vi "Show Recipe.vi"(8 "error in (no error)":errorcluster, 10 "List Index":i32, 11 "Main Window in":refnum<class "Main Window.lvclass">) -> (0 "error out":errorcluster, 3 "Main Window out":refnum<class "Main Window.lvclass">)   [LabVIEW 2021, in "Recipe.lvlib" / "Main Window.lvclass"]
uses:
  Main Window.lvclass
  Main Window.lvclass/Main Window.ctl
  <vilib>/MGI/Panel Manager/Panel Actor/Panel Actor Messages/Show Panel Msg/Show Panel Msg.lvclass
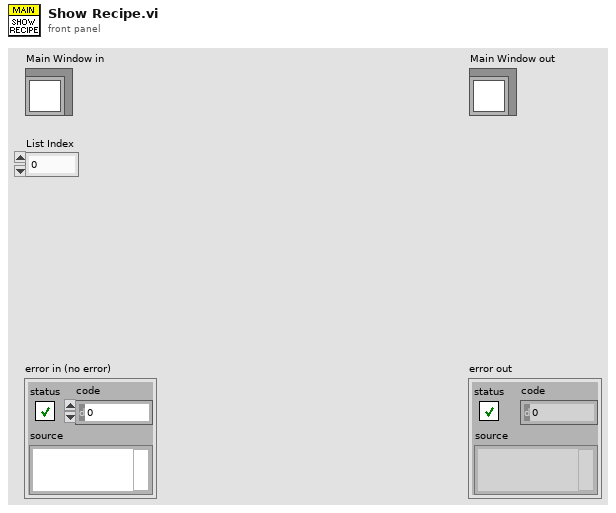
[diagram p1: front panel]
types:
  T1 = map{string, refnum<class "Message Enqueuer.lvclass">}
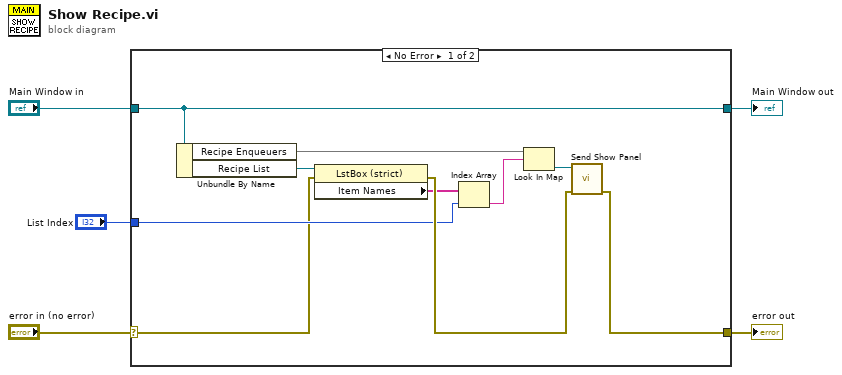
[diagram p0: block diagram]
diagram:
  n1 = case shown="No Error" "error in (no error)" {
    selector: "error in (no error)" -> [w10 w17]
    tunnel: [w6 w17] -> w4
    tunnel: [w14 w16] -> w2
    tunnel: "Main Window in" -> [w14 w16]
    tunnel: "List Index" -> [w11 _]
    frame No Error {
      n2 = Unbundle By Name(w14) -> ("Recipe Enqueuers"=w9:T1, "Recipe List"=w13:refnum<vi>)
      n3 = property class="LstBox (strict)"(reference=w13, error in=w10) -> (error out=w15:errorcluster, "Item Names"=w12:string[])  [unwired: 1 out]
      n4 = Index Array(array=w12, index=w11) -> (element=w8:string)
      n5 = Look In Map(map=w9, key=w8) -> (value=w7:refnum<class "Message Enqueuer.lvclass">)  [unwired: 1 in, 1 out]
      n6 = call <vilib>:"Send Show Panel.vi"("Error In"=w15, "Message Enqueuer in"=w7) -> ("Error Out"=w6:errorcluster)  [unwired: 8 in, 1 out]
    }
    frame Error {
    }
  }
  "error out" <- w4
  "Main Window out" <- w2
